vi "所有告警信息组合.vi"(9 "x 3":i32=300001, 10 "x 2":i32=200001, 11 "x":i32=100001) -> (1 "输出结果3":string[][](array[string]), 2 "输出结果2":string[][](array[string]), 3 "输出结果1":string[][](array[string]))   [LabVIEW 2016, in "Alarm interface.lvlib"]
uses:
  Alarm interface.lvlib
  <userlib>/_OpenG.lib/array/array.llb/Remove Duplicates from 1D Array (String)__ogtk.vi
panel:
  in  "选项卡控件":T1(tab)
  in  "营养盐报警常量":T2=[["1", "100007", "缺试剂告警", "1、建议排查管路是否异常\n2、供电情况是否正常"], ["2", "100008", "缺水样告警", "1、配水箱内无水样；\n2、配水箱到模块的管路气密性不佳；\n3、注射泵水样阀口堵塞；\n4、注射泵阀过载或丝杆无动作。"], ["3", "100009", "缺纯水告警", "1、建议排查管路是否异常\n2、供电情况是否正常"], ["4", "100010", "缺标液告警", "1、注射泵水样阀口堵塞；\n2、注射泵阀过载或丝杆无动作。"], ["5", "200007", "仪表漏液告警", "1、建议排查管路是否异常\n2、供电情况是否正常"], ["6", "100011", "标定异常告警", "1、建议排查管路是否异常\n2、供电情况是否正常"], ["7", "4", "超量程告警", "1、建议排查管路是否异常\n2、供电情况是否正常"], ["8", "200008", "加热告警", "检查温度传感器、检查加热片是否损坏或脱落、检查加热模块与电路板接线是否正常、检查固件是否匹配"], ["9", "100051", "低试剂预警", "1、建议排查管路是否异常\n2、供电情况是否正常"], ["10", "1", "超上限告警", "1、建议排查管路是否异常\n2、供电情况是否正常"], ["11", "2", "超下限告警", "1、建议排查管路是否异常\n2、供电情况是否正常"], ["12", "100012", "其他告警", "1、建议排查管路是否异常\n2、供电情况是否正常"], ["13", "100028", "滴定异常告警", "1、建议排查管路是否异常\n2、供电情况是否正常"], ["14", "100069", "电极异常告警", "1、建议排查管路是否异常\n2、供电情况是否正常"], ["15", "3", "量程切换告警", "1、建议排查管路是否异常\n2、供电情况是否正常"], ["16", "100070", "参数设置告警", "1、建议排查管路是否异常\n2、供电情况是否正常"], ["17", "100071", "pH电极电位异常", "1、建议排查管路是否异常\n2、供电情况是否正常"], ["18", "100072", "电导率电极异常", "1、建议排查管路是否异常\n2、供电情况是否正常"], ["19", "100073", "浊度光度异常", "1、建议排查管路是否异常\n2、供电情况是否正常"], ["20", "100074", "溶解氧电极异常", "1、建议排查管路是否异常\n2、供电情况是否正常"], ["21", "100075", "溶解氧光强异常", "1、建议排查管路是否异常\n2、供电情况是否正常"], ["22", "100076", "温度异常告警", "1、建议排查管路是否异常\n2、供电情况是否正常"], ["23", "100077", "pH异常告警", "1、建议排查管路是否异常\n2、供电情况是否正常"], ["24", "100078", "溶解氧异常告警", "1、建议排查管路是否异常\n2、供电情况是否正常"], ["25", "100079", "电导率异常告警", "1、建议排查管路是否异常\n2、供电情况是否正常"], ["26", "100080", "浊度异常告警", "1、建议排查管路是否异常\n2、供电情况是否正常"], ["27", "100081", "叶绿素a异常告警", "1、建议排查管路是否异常\n2、供电情况是否正常"], ["28", "100082", "藻密度异常告警", "1、建议排查管路是否异常\n2、供电情况是否正常"], ["29", "100083", "蓝绿藻异常告警", "1、建议排查管路是否异常\n2、供电情况是否正常"], ["30", "100084", "ORP异常告警", "1、建议排查管路是否异常\n2、供电情况是否正常"], ["31", "100085", "氨氮异常告警", "1、建议排查管路是否异常\n2、供电情况是否正常"], ["32", "100086", "清洁刷异常告警", "1、建议排查管路是否异常\n2、供电情况是否正常"], ["33", "100087", "SD卡异常告警", "1、建议排查管路是否异常\n2、供电情况是否正常"], ["34", "100088", "蓝牙异常告警", "1、建议排查管路是否异常\n2、供电情况是否正常"], ["35", "100089", "WIFI异常告警", "1、建议排查管路是否异常\n2、供电情况是否正常"], ["36", "100013", "缺流程告警", "流程未写入、芯片异常，未存储"], ["37", "100014", "芯片存储异常告警", "固件异常"], ["38", "100015", "缺公式告警", "公式未写入、芯片异常，未存储"], ["40", "6", "光值过低告警", "1、检查比色皿是否污染严重；\n2、检查水体浊度是否过高。"], ["41", "5", "光值过高告警", "检查光强是否漂移"], ["42", "100017", "温度探头接线异常告警", "1、建议排查管路是否异常\n2、供电情况是否正常"], ["43", "100018", "温度探头未嵌入凹槽或消解模", "1、建议排查管路是否异常\n2、供电情况是否正常"], ["44", "100019", "温度探头功率过大告警", "1、建议排查管路是否异常\n2、供电情况是否正常"], ["61", "100008", "缺水样告警", "1、建议排查管路是否异常\n2、供电情况是否正常"], ["62", "100010", "缺标样告警", "1、建议排查管路是否异常\n2、供电情况是否正常"], ["63", "100046", "缺零点核查样告警", "1、建议排查管路是否异常\n2、供电情况是否正常"], ["64", "100047", "缺跨度核查样告警", "1、建议排查管路是否异常\n2、供电情况是否正常"], ["65", "100048", "缺空白样告警", "1、建议排查管路是否异常\n2、供电情况是否正常"], ["66", "100049", "缺平行样告警", "1、建议排查管路是否异常\n2、供电情况是否正常"], ["67", "100050", "缺加标样告警", "1、建议排查管路是否异常\n2、供电情况是否正常"], ["70", "100051", "缺试剂A", "1、建议排查管路是否异常\n2、供电情况是否正常"], ["71", "100052", "缺试剂B", "1、建议排查管路是否异常\n2、供电情况是否正常"], ["81", "100053", "水样余量过低，请及时维护", "1、建议排查管路是否异常\n2、供电情况是否正常"], ["82", "100054", "标液余量过低，请及时维护", "1、建议排查管路是否异常\n2、供电情况是否正常"], ["83", "100055", "零点样余量过低，请及时维护", "1、建议排查管路是否异常\n2、供电情况是否正常"], ["84", "100056", "跨度样余量过低，请及时维护", "1、建议排查管路是否异常\n2、供电情况是否正常"], ["85", "100057", "空白样余量过低，请及时维护", "1、建议排查管路是否异常\n2、供电情况是否正常"], ["86", "100058", "平行样余量过低，请及时维护", "1、建议排查管路是否异常\n2、供电情况是否正常"], ["87", "100059", "加标样余量过低，请及时维护", "1、建议排查管路是否异常\n2、供电情况是否正常"], ["90", "100060", "试剂A余量过低，请及时维护", "1、建议排查管路是否异常\n2、供电情况是否正常"], ["91", "100061", "试剂B余量过低，请及时维护", "1、建议排查管路是否异常\n2、供电情况是否正常"], ["99", "100023", "注射泵配置异常告警", "代码99：检查流程是否错误，查询注射泵配置信息是否不匹配"], ["103", "100020", "注射泵供电异常告警", "代码103：注射泵未初始化，检查电压是否正常"], ["105", "100021", "注射泵丝杆过载告警", "代码105：检查丝杆是否生锈、检查注射器阻力是否正常、检查注射泵自检是否正常"], ["106", "100022", "注射泵阀头切换过载告警", "代码106：检查阀口是否堵塞、检查多通阀转子接触面是否黏结"], ["250", "100062", "请注意查看溶液或试剂余量并", "1、建议排查管路是否异常\n2、供电情况是否正常"], ["253", "100063", "旋转阀通讯异常告警", "1、建议排查管路是否异常\n2、供电情况是否正常"], ["254", "100025", "光谱仪通讯异常告警", "1、建议排查管路是否异常\n2、供电情况是否正常"], ["255", "100024", "注射泵通讯异常告警", "代码255：检查注射泵与电路板通讯是否正常"], ["500", "100090", "试剂不足", "试剂不足，请及时补充试剂"], ["501", "100091", "试剂余量检测异常", "请查询固件流程是否匹配，试剂是否有倒灌现象"]]
  in  "V2CODMn报警常量":T3=[["1", "100092", "电极异常", "1.ORP电极线路连接异常\n2.ORP传感器故障\n3.采集ORP的PLC模拟量采集模块故障"], ["2", "100093", "温控器故障", "1.PT100线路连接异常\n2.PT100传感器故障\n3.采集温度的PLC模拟量采集模块故障"], ["3", "200009", "加热故障", "1.PT100线路连接异常\n2.PT100传感器故障\n3.采集温度的PLC模拟量采集模块故障\n1.缺水样导致\n2.PT100异常"], ["4", "100094", "高锰酸钾异常", "1.缺高锰酸钾试剂\n2.检测水样浓度过高"], ["5", "100095", "草酸钠异常", "1.缺草酸钠试剂\n2.高锰酸钾配制浓度错误"], ["6", "100096", "测量错误", "1.检查其他异常告警"], ["7", "100097", "校标错误", "1.检查其他异常告警"], ["8", "100098", "进水样超量程", "1.进水样超过最大体积"], ["9", "100099", "排液阀故障", "1.检查排液阀\n2.检查排液管上的液位传感器"], ["10", "100100", "60分钟超时报警", "1.水样浓度过高导致超时\n2.反滴定速度过慢导致超时"], ["11", "100101", "进样无液体报警", "1.检查进样泵\n2.检查进样管上的液位传感器"]]
  in  "新CODMn报警常量":T4=[["1", "100007", "缺试剂告警", "1、是否缺试剂，及时补充试剂\n2、对应的试剂阀口堵塞，及时清理并更换连接头。\n3、管路气密性不佳\n4、检查传感器与电路板连接、查看传感器光值是否异常"], ["2", "100008", "缺水样告警", "1、配水箱内无水样\n2、对应的水样阀口堵塞或者三通阀坏掉，不能正常切换\n3、往复式注射泵异常，或者管路气密性不佳\n4、检查水样传感器与电路板连接、查看水样传感器光值是否异常"], ["3", "100009", "缺纯水告警", "1、建议排查管路是否异常\n2、供电情况是否正常"], ["4", "100010", "缺标液告警", "1、注射泵水样阀口堵塞；\n2、注射泵阀过载或丝杆无动作。"], ["5", "200007", "仪表漏液告警", "1、建议排查管路是否异常\n2、供电情况是否正常"], ["6", "100011", "标定异常告警", "1、建议排查管路是否异常\n2、供电情况是否正常"], ["7", "4", "超量程告警", "1、建议排查管路是否异常\n2、供电情况是否正常"], ["8", "200008", "加热告警", "检查温度传感器、检查加热片是否损坏或脱落、检查加热模块与电路板接线是否正常、检查固件是否匹配"], ["9", "100051", "低试剂预警", "1、建议排查管路是否异常\n2、供电情况是否正常"], ["10", "1", "超上限告警", "1、建议排查管路是否异常\n2、供电情况是否正常"], ["11", "2", "超下限告警", "1、建议排查管路是否异常\n2、供电情况是否正常"], ["12", "100012", "其他告警", "1、建议排查管路是否异常\n2、供电情况是否正常"], ["13", "100028", "滴定异常告警", "1、配水箱内无水样；\n2、配水箱到模块的管路气密性不佳；\n3、注射泵水样阀口堵塞；\n4、注射泵阀过载或丝杆无动作。"], ["14", "100069", "电极异常告警", "1、建议排查管路是否异常\n2、供电情况是否正常"], ["15", "3", "量程切换告警", "1、建议排查管路是否异常\n2、供电情况是否正常"], ["16", "100070", "参数设置告警", "1、建议排查管路是否异常\n2、供电情况是否正常"], ["17", "100071", "pH电极电位异常", "1、建议排查管路是否异常\n2、供电情况是否正常"], ["18", "100072", "电导率电极异常", "1、建议排查管路是否异常\n2、供电情况是否正常"], ["19", "100073", "浊度光度异常", "1、建议排查管路是否异常\n2、供电情况是否正常"], ["20", "100074", "溶解氧电极异常", "1、建议排查管路是否异常\n2、供电情况是否正常"], ["21", "100029", "缺高锰酸钾告警", "1、建议排查管路是否异常\n2、供电情况是否正常"], ["22", "100030", "缺草酸钠告警", "1、建议排查管路是否异常\n2、供电情况是否正常"], ["23", "100031", "缺硫酸告警", "1、建议排查管路是否异常\n2、供电情况是否正常"], ["24", "100078", "溶解氧异常告警", "1、建议排查管路是否异常\n2、供电情况是否正常"], ["25", "100079", "电导率异常告警", "1、建议排查管路是否异常\n2、供电情况是否正常"], ["26", "100080", "浊度异常告警", "1、建议排查管路是否异常\n2、供电情况是否正常"], ["27", "100081", "叶绿素a异常告警", "1、建议排查管路是否异常\n2、供电情况是否正常"], ["28", "100082", "藻密度异常告警", "1、建议排查管路是否异常\n2、供电情况是否正常"], ["29", "100083", "蓝绿藻异常告警", "1、建议排查管路是否异常\n2、供电情况是否正常"], ["30", "100084", "ORP异常告警", "1、建议排查管路是否异常\n2、供电情况是否正常"], ["31", "100085", "氨氮异常告警", "1、建议排查管路是否异常\n2、供电情况是否正常"], ["32", "100086", "清洁刷异常告警", "1、建议排查管路是否异常\n2、供电情况是否正常"], ["33", "100087", "SD卡异常告警", "1、建议排查管路是否异常\n2、供电情况是否正常"], ["34", "100088", "蓝牙异常告警", "1、建议排查管路是否异常\n2、供电情况是否正常"], ["35", "100089", "WIFI异常告警", "1、建议排查管路是否异常\n2、供电情况是否正常"], ["36", "100013", "缺流程告警", "流程未写入、芯片异常，未存储"], ["37", "100014", "芯片存储异常告警", "固件异常"], ["38", "100015", "缺公式告警", "公式未写入、芯片异常，未存储"], ["39", "100032", "ORP值异常告警", "请检查是否缺水样、ORP电极与电路板连接、更换ORP电极、更换ORP电极采集板，电路板排查"], ["40", "100033", "A值异常告警", "（1）水样浓度过高，需切换到高量程测试。\n（2）缺高锰酸钾或硫酸，可通过试剂报警判断。\n（3）高锰酸钾过期，浓度降低。\n（4）试剂管路或者阀口气密性不好，有空气进入。\n（5）九通注射泵故障，没有正常进样。\n（6）ORP电极故障，无法正常工作。（可通过单步启动测试，观察电极读数有无明显变化）"], ["41", "100034", "B值异常告警", "（1）缺草酸钠或硫酸，可通过试剂报警判断。\n（2）草酸钠过期，浓度降低较多。\n（3）试剂管路或者阀口气密性不好，有空气进入。\n（4）九通注射泵故障，没有正常进样。\n（5）ORP电极故障，无法正常工作。（可通过单步启动测试，观察电极读数有无明显变化）"], ["42", "100035", "环境温度传感器告警", "检查温度传感器与电路板连接，更换温度传感器排查"], ["43", "100036", "注射器保温温度异常告警", "检查温度传感器与电路板连接，更换温度传感器排查"], ["44", "100037", "注射器保温加热超时告警", "检查加热保温圈是否损坏或脱落、加热保温圈与电路板连接、温度传感器是否脱落"], ["96", "100102", "高锰酸钾试剂余量过低，请及时维护", "1、建议排查管路是否异常\n2、供电情况是否正常"], ["97", "100103", "草酸钠试剂余量过低，请及时维护", "1、建议排查管路是否异常\n2、供电情况是否正常"], ["98", "100104", "硫酸试剂余量过低，请及时维护", "1、建议排查管路是否异常\n2、供电情况是否正常"], ["99", "100023", "注射泵配置异常告警", "1、建议排查管路是否异常\n2、供电情况是否正常"], ["103", "100020", "注射泵供电异常告警", "代码103：注射泵未初始化，检查电压是否正常"], ["105", "100021", "注射泵管路阻塞告警", "代码105：检查丝杆是否生锈、检查注射器阻力是否正常、检查注射泵自检是否正常"], ["106", "100022", "注射泵阀头切换过载告警", "代码106：检查阀口是否堵塞、检查多通阀转子接触面是否黏结"], ["250", "100044", "偏心轮运行超时告警", "运行超时告警，检查该器件是否正常运转，或者运转非常缓慢，更换器件排查"], ["253", "100105", "加热温度超限告警", "检查温度传感器与电路板连接、检查是否缺水样"], ["254", "100106", "加热或者降温超时告警", "1、建议排查管路是否异常\n2、供电情况是否正常"], ["255", "100024", "注射泵通讯异常告警", "代码255：检查注射泵与电路板通讯是否正常"]]
  in  "动力环境报警常量":T5=[["1", "100001", "市电异常", "1、建议排查通信是否正常\n2、供电情况是否正常"], ["2", "100002", "UPS异常", "1、建议排查通信是否正常\n2、供电情况是否正常"], ["3", "100003", "蓄电池异常", "1、建议排查通信是否正常\n2、供电情况是否正常"], ["4", "100004", "空调异常", "1、建议排查通信是否正常\n2、供电情况是否正常"], ["5", "200001", "温湿度异常", "1、建议排查通信是否正常\n2、供电情况是否正常\n3、环境温湿度超上限"], ["6", "200002", "移位告警", "1、建议排查通信是否正常\n2、供电情况是否正常\n3、位置偏移"], ["7", "200003", "烟雾告警", "1、建议排查通信是否正常\n2、供电情况是否正常\n3、检测到浓烟"], ["8", "200004", "振动告警", "1、建议排查通信是否正常\n2、供电情况是否正常\n3、检测到振动"], ["9", "200005", "红外入侵告警", "1、建议排查通信是否正常\n2、供电情况是否正常\n3、检测到入侵"], ["10", "200006", "漏水告警", "1、建议排查通信是否正常\n2、供电情况是否正常\n3、检测到漏水"]]
  in  "质控单元报警常量":T6=[["1", "100066", "液位异常告警", "1、建议排查通信是否正常\n2、供电情况是否正常"], ["2", "100067", "柱塞泵故障告警", "1、建议排查通信是否正常\n2、供电情况是否正常"], ["3", "100068", "流程中断告警", ""]]
  out "组合数组":string[][](array[string])
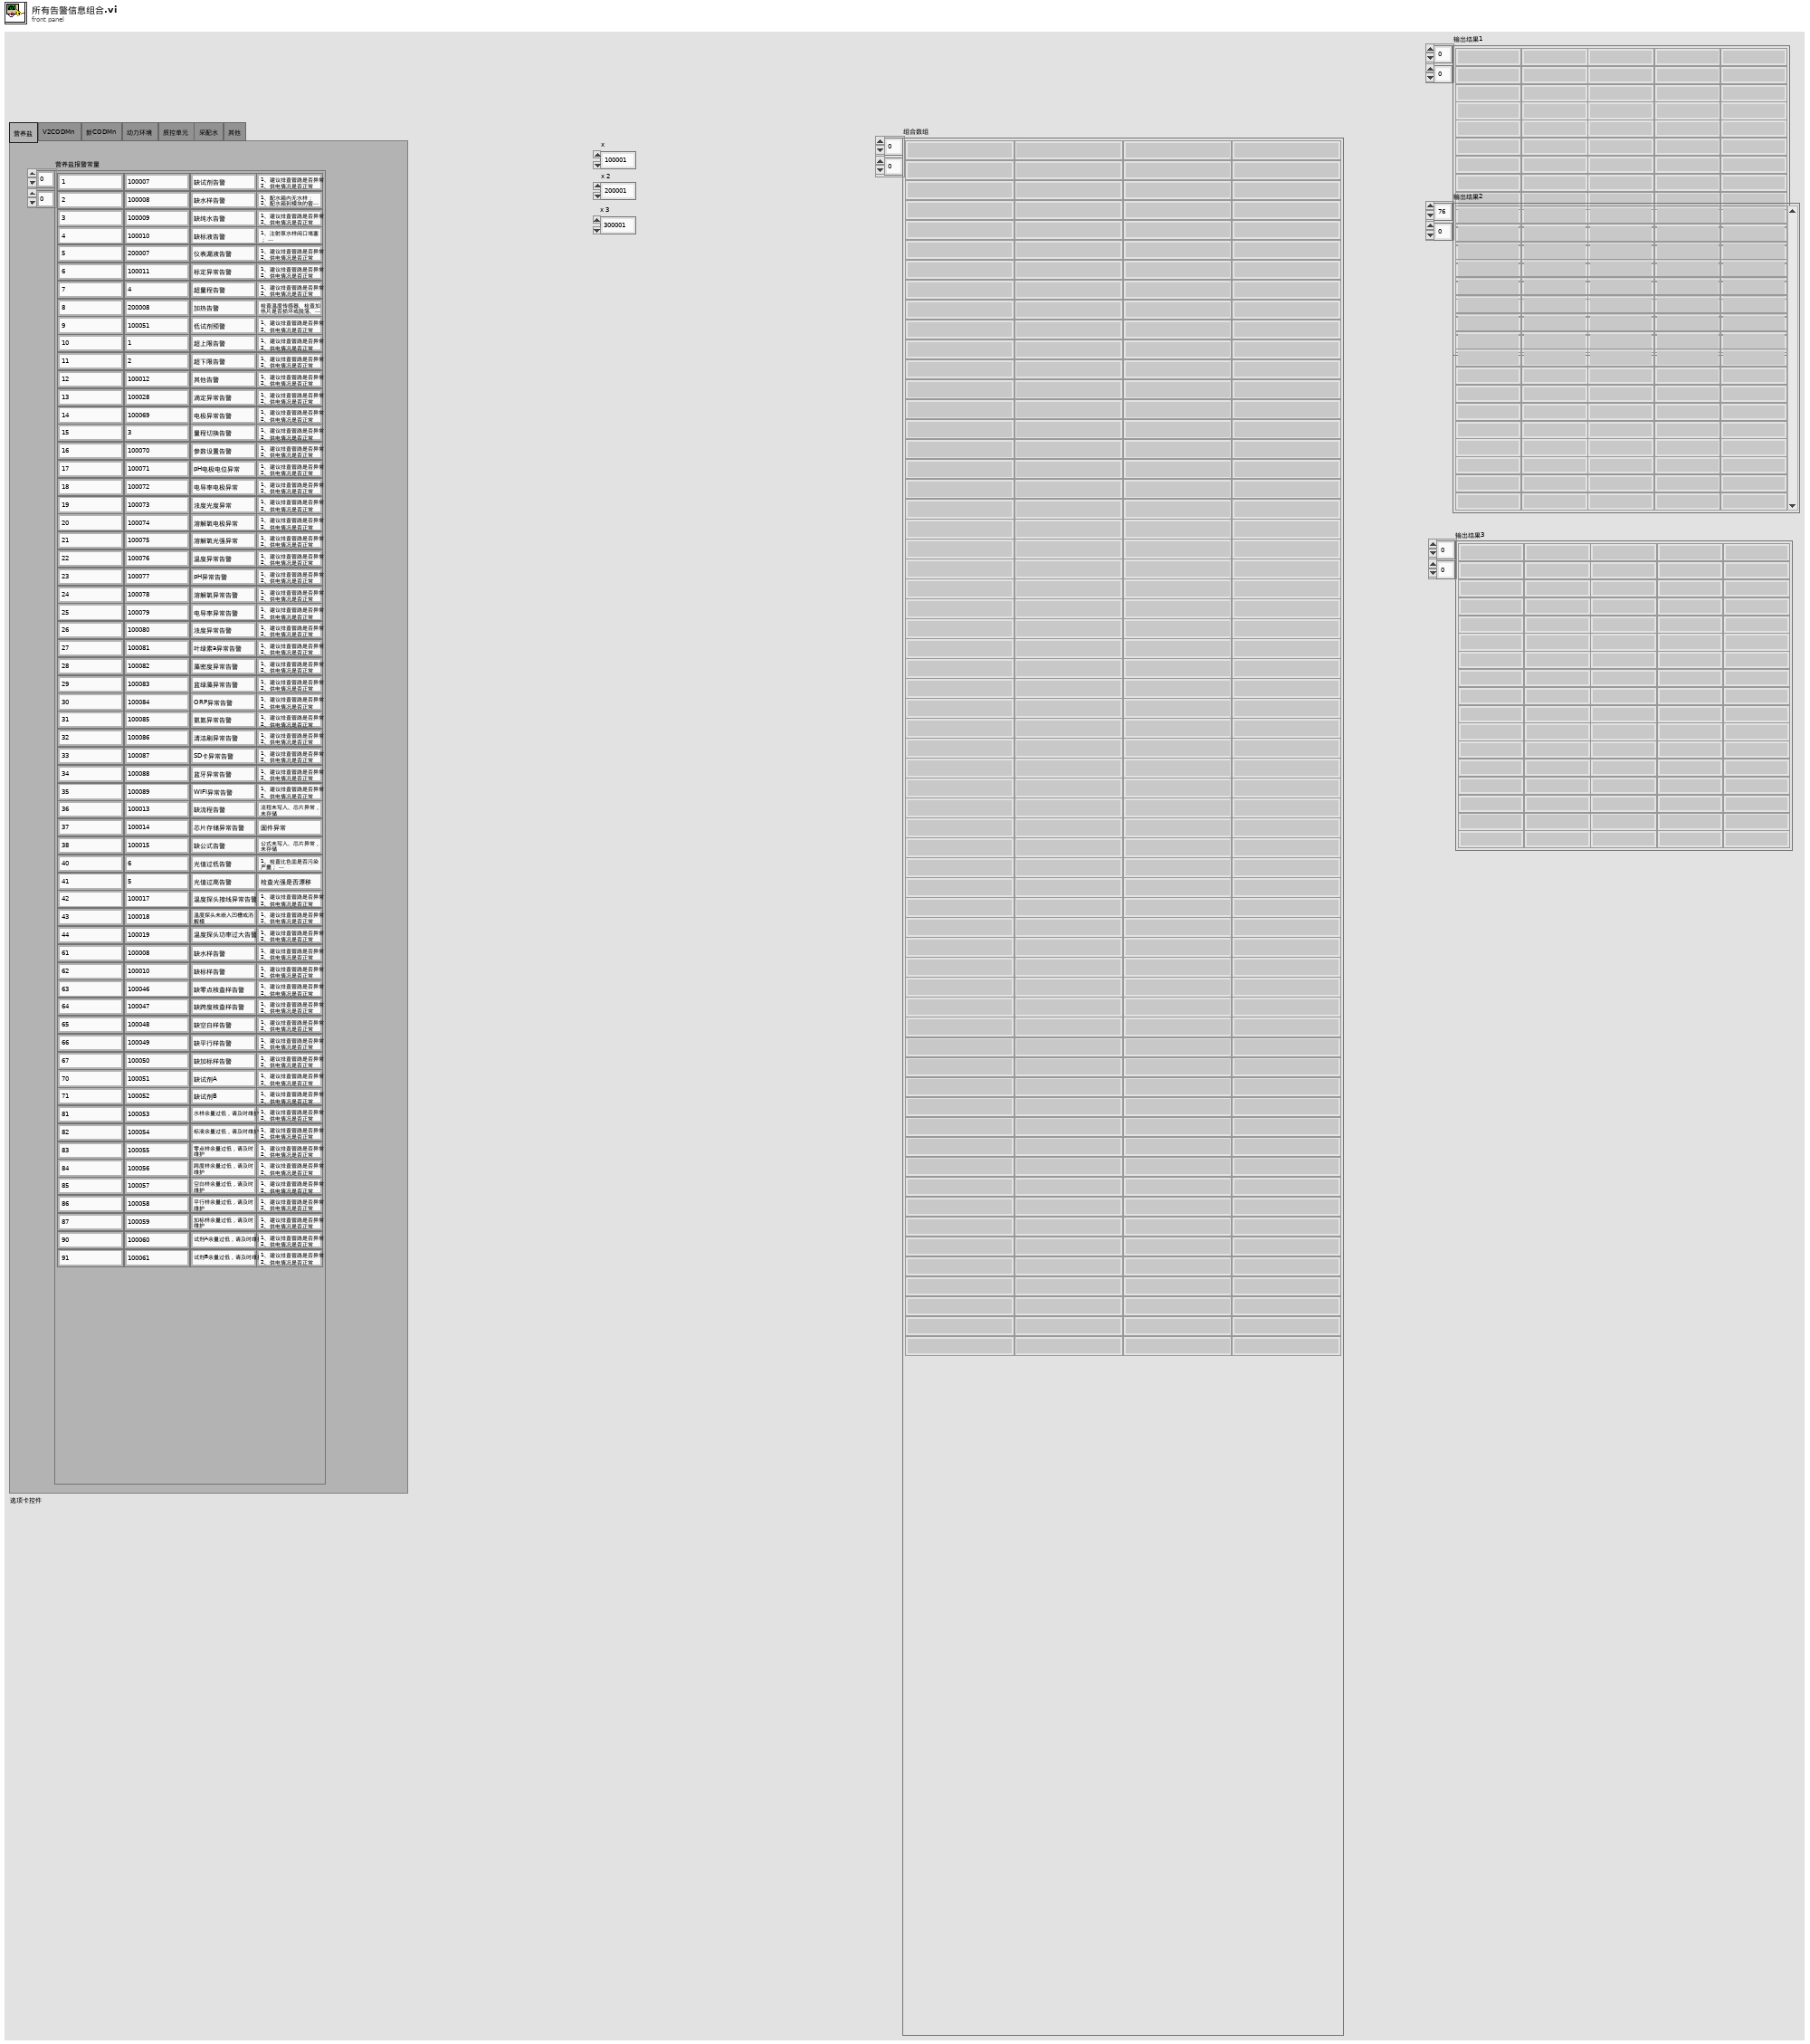
[diagram p1: front panel]
types:
  T1 = enum32{"营养盐", "V2CODMn", "新CODMn", "动力环境", "质控单元", "采配水", "其他"}
  T2 = typedef "Alarm interface.lvlib/营养盐报警.ctl" = string[][]
  T3 = typedef "Alarm interface.lvlib/V2CODMn报警.ctl" = string[][]
  T4 = typedef "Alarm interface.lvlib/新CODMn报警.ctl" = string[][]
  T5 = typedef "Alarm interface.lvlib/动力环境报警.ctl" = string[][]
  T6 = typedef "Alarm interface.lvlib/质控单元报警.ctl" = string[][]
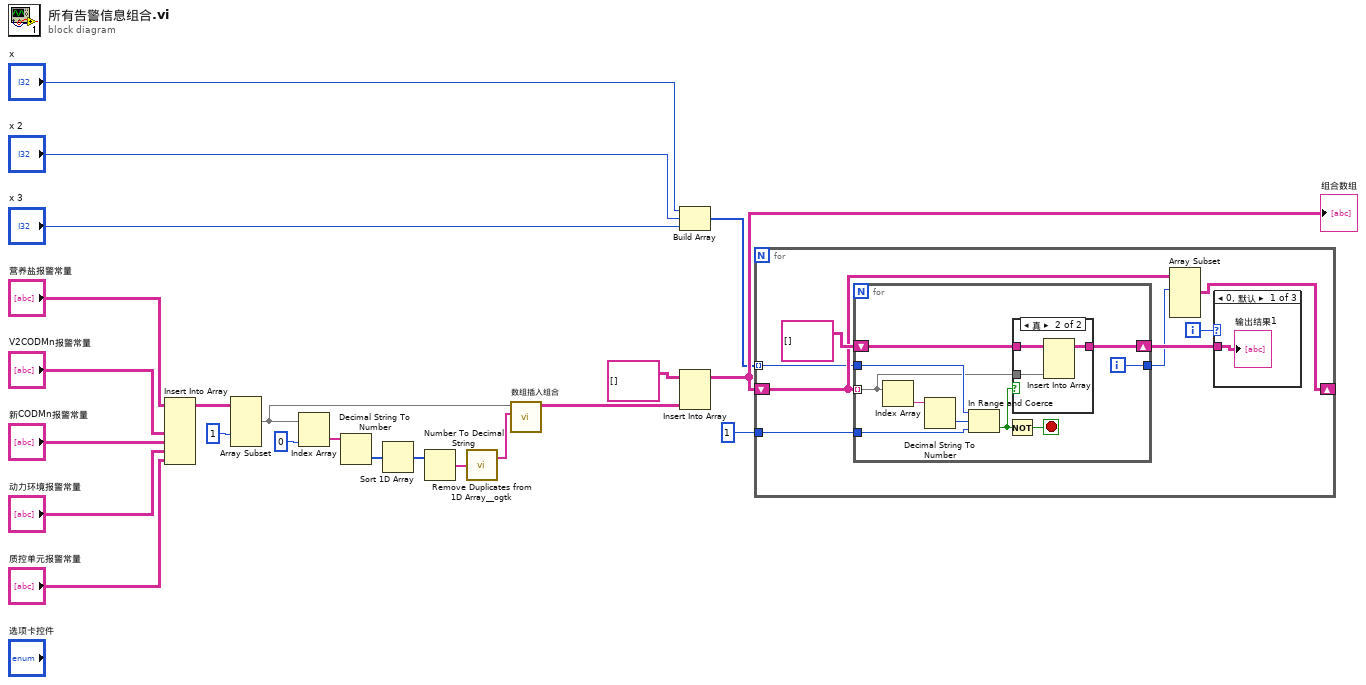
[diagram p0: block diagram]
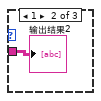
[diagram p2: hidden frame]
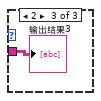
[diagram p3: hidden frame]
diagram:
  n1 = Insert Into Array(array="营养盐报警常量", new element #1="V2CODMn报警常量", new element #2="新CODMn报警常量", new element #3="动力环境报警常量", new element #4="质控单元报警常量") -> (w12:T2)  [unwired: 2 in]
  n2 = Array Subset(array=w12, index (col)=1 ("索引")) -> (w15:T2)  [unwired: 3 in]
  n3 = Index Array(array=w15, index (col)=0 ("禁用的索引 (列)")) -> (element=w18:string[])  [unwired: 1 in]
  n4 = Decimal String To Number(string=w18) -> (number=w19:i32[])  [unwired: 2 in, 1 out]
  n5 = Sort 1D Array(array=w19) -> (sorted array=w20:i32[])
  n6 = Number To Decimal String(number=w20) -> (decimal integer string=w14:string[])  [unwired: 1 in]
  n7 = call-poly <userlib>:"Remove Duplicates from 1D Array__ogtk.vi"("Input Array"=w14) -> ("Output Array"=w13:string[])  [unwired: 1 out]
  n8 = call "数组插入组合.vi"("排序后的一维数组"=w13, "输入数组"=w15) -> ("输出结果"=w16:string[][])  [unwired: 9 in]
  n9 = Build Array("x", "x 2", "x 3") -> (w6:i32[])
  n10 = Insert Into Array(array=string[][] [] ("输出结果"), new element=w16) -> (w10:string[][])  [unwired: 2 in]
  "组合数组" <- w10
  n11 = for {
    tunnel: 1 ("x") -> [w30]
    shift-right: [w26] -> _
    shift-left: w10 -> [w25]
    tunnel: w6 -> [w23] mode=indexing
    i -> [w24]
    n12 = for {
      tunnel: w25 -> [w39] mode=indexing
      tunnel: w30 -> [w40]
      tunnel: w23 -> [w41]
      shift-right: [w35] -> w29
      shift-left: string[][] [] ("输出结果 2") -> [w36]
      tunnel: [w34] -> w27
      i -> [w34]
      stop <- w37 stop-if-true
      n13 = Index Array(array=w39) -> (element=w43:string)  [unwired: 1 in]
      n14 = Decimal String To Number(string=w43) -> (number=w42:i32)  [unwired: 2 in, 1 out]
      n15 = In Range and Coerce(upper limit=w41, x=w42, lower limit=w40) -> (In Range?=w38:bool)  [unwired: 1 out]
      n16 = Not(x=w38) -> (.not. x?=w37:bool)
      n17 = case shown="真" w38 {
        tunnel: w39 -> [_ w46]
        tunnel: [w44 w45] -> w35
        tunnel: w36 -> [w44 w47]
        frame False {
        }
        frame True {
          n18 = Insert Into Array(array=w47, new element=w46) -> (w45:string[][])  [unwired: 2 in]
        }
      }
    }
    n19 = Array Subset(array=w25, index (row)=w27) -> (w26:string[][])  [unwired: 3 in]
    n20 = case shown="0, 默认" w24 {
      tunnel: w29 -> [w31 w32 w33]
      frame 0, Default {
        "输出结果1" <- w31
      }
      frame 1 {
        "输出结果2" <- w32
      }
      frame 2 {
        "输出结果3" <- w33
      }
    }
  }
